vi "clip_max_search.vi"(0 "input cluster":T1, 1 "Channel":i32, 2 "vclip":i32, 5 "Vatt init":i32=4095, 7 "Boolean":bool=TRUE, 9 "Voltage value":dbl=0.05, 11 "error out 2":errorcluster) -> (4 "output cluster":T1={"AWG VISA"="81160A", "Oscilloscope  VISA "="", "Integration Board IP"="172.16.7.43", "connection ID"=refnum, "report out"=refnum, "report file path"=path ""}, 6 "Vatt init":i32, 8 "vclip":i32, 10 "L1 value":i32, 15 "error out":errorcluster)   [LabVIEW 2009]
uses:
  <vilib>/Utility/NIReport.llb/NI_report.lvclass
  <instrlib>/Agilent 81150/Agilent 81150.lvlib
panel:
  in  "vclip_fi":i32
  out "L1 vs vatt":cluster{i32[], i32[]}(graph)
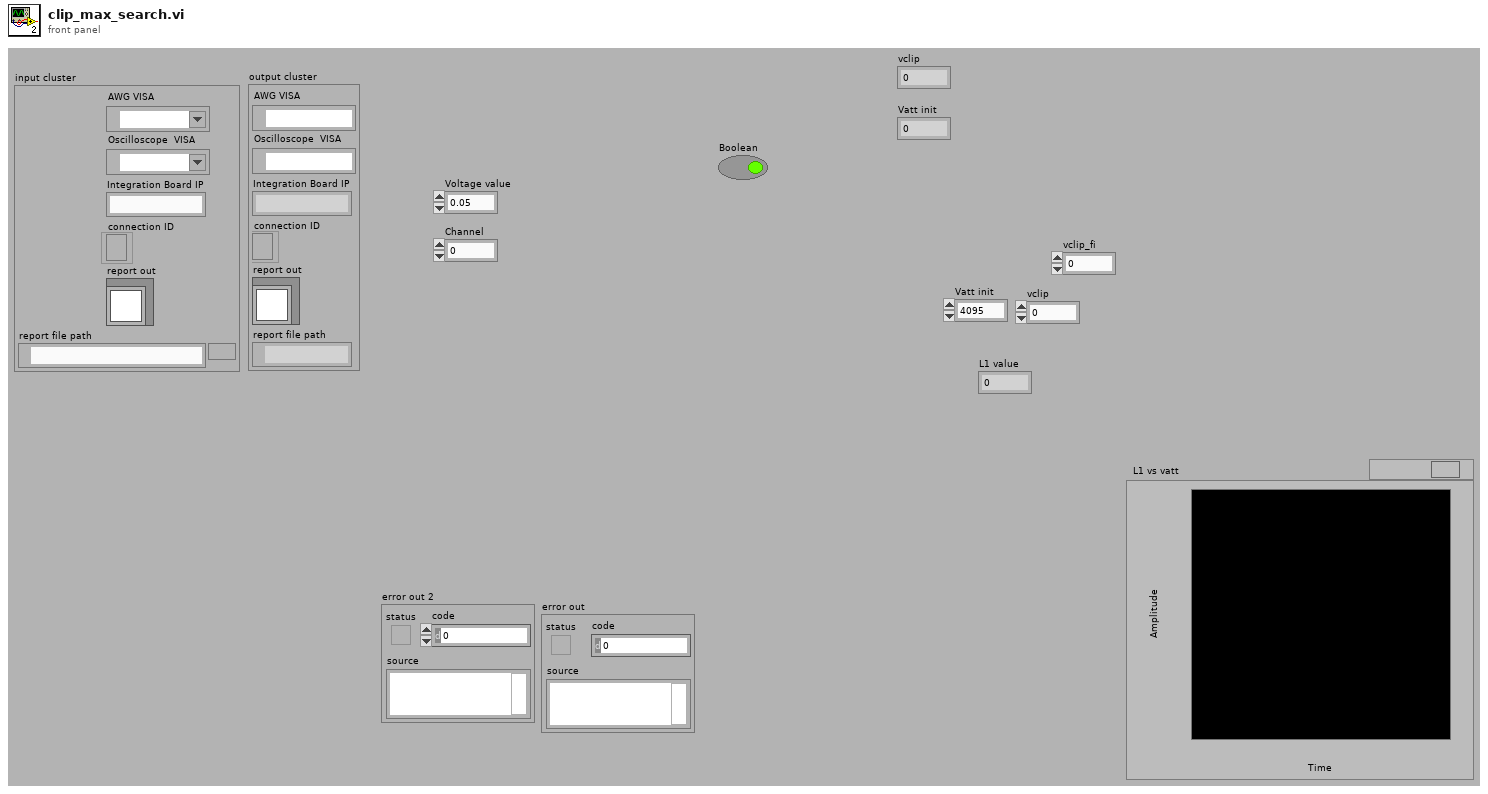
[diagram p1: front panel]
types:
  T1 = cluster{"AWG VISA":refnum<visa-resource-name>, "Oscilloscope  VISA ":refnum<visa-resource-name>, "Integration Board IP":string, "connection ID":refnum<k5>, "report out":refnum<class "NI_report.lvclass">, "report file path":path}
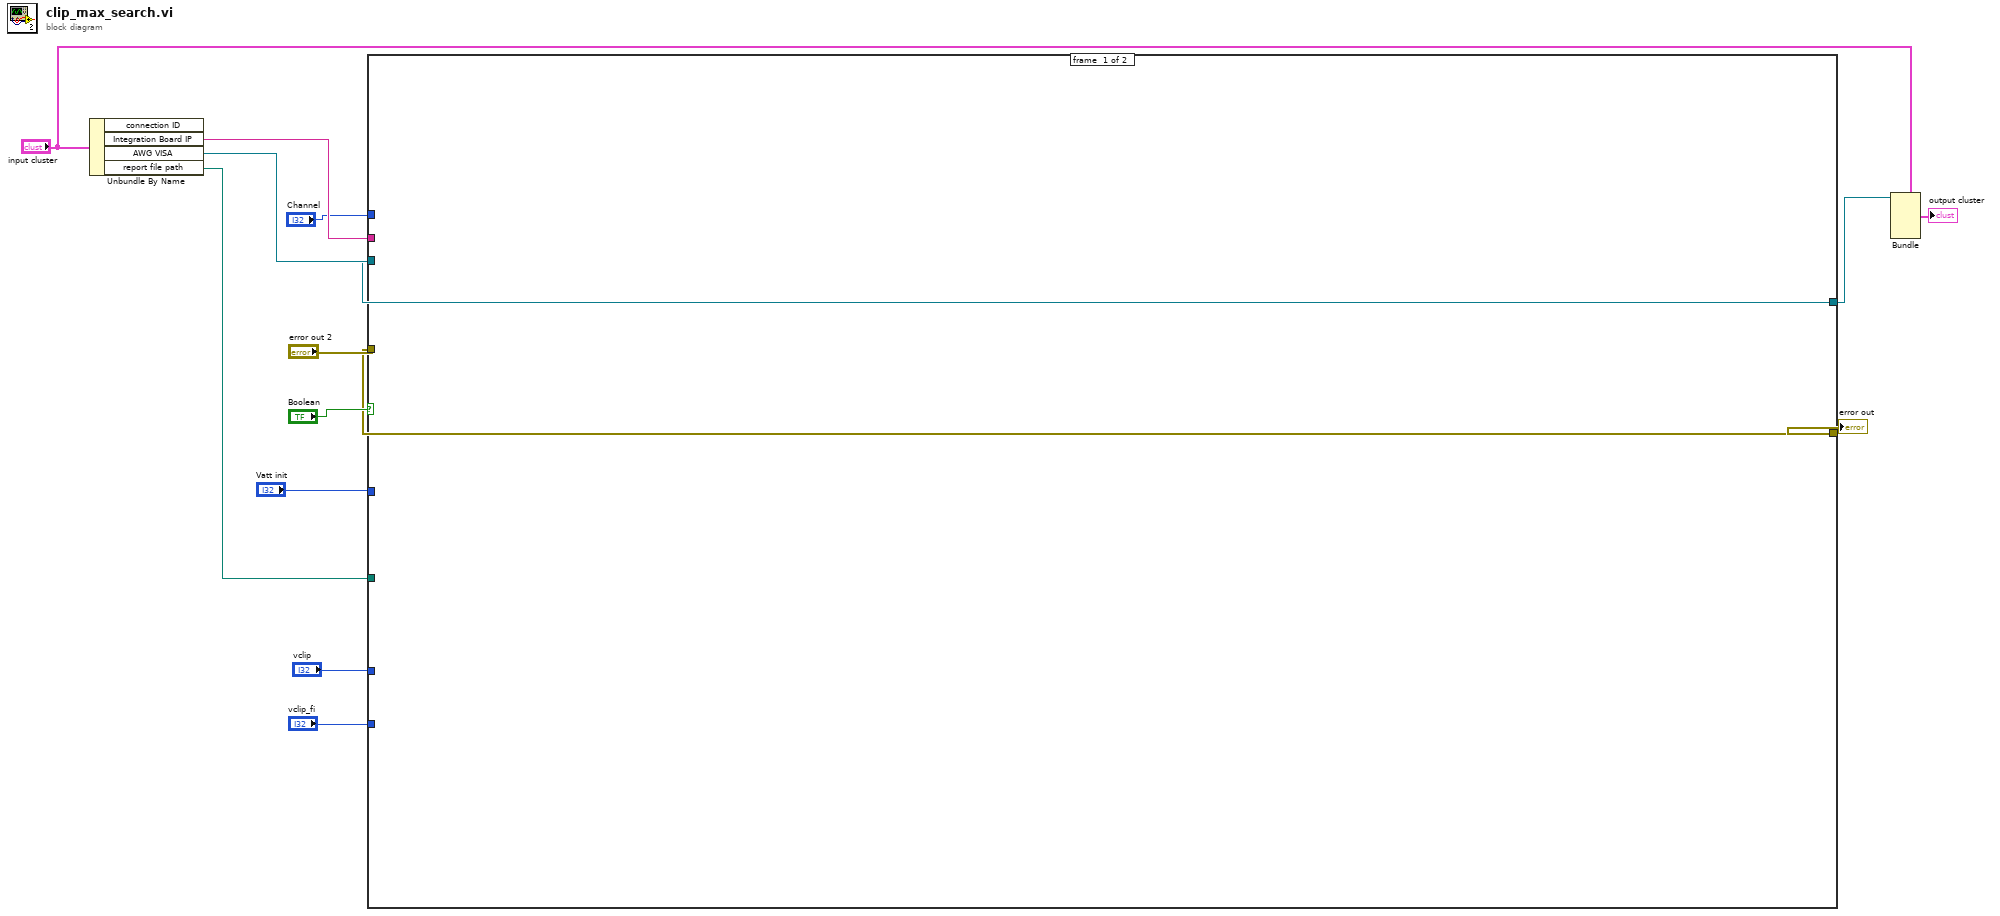
[diagram p0: block diagram]
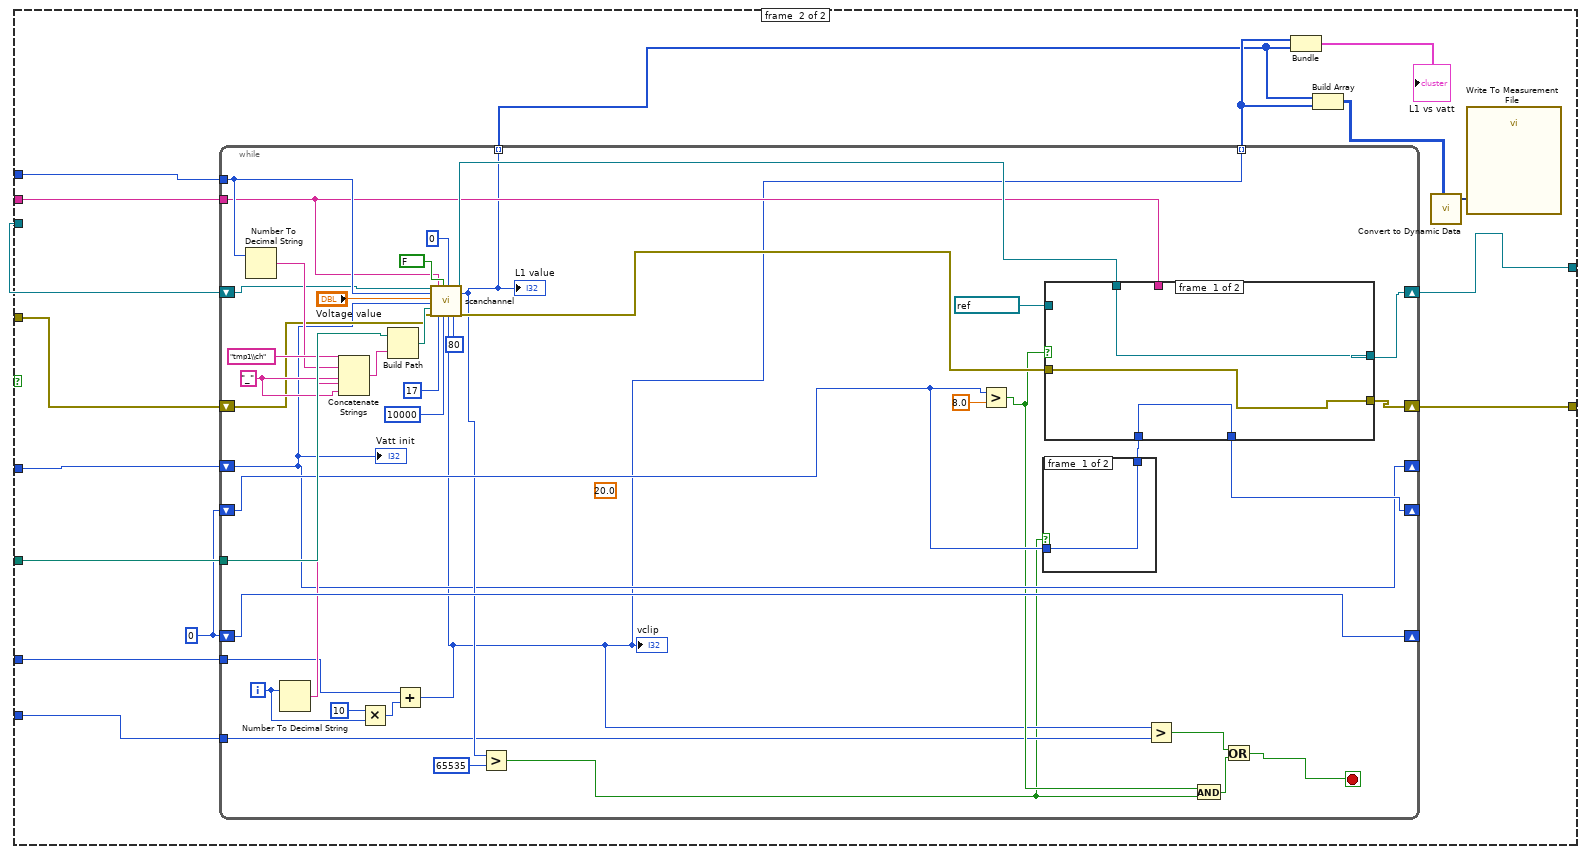
[diagram p2: hidden frame]
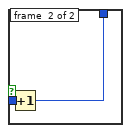
[diagram p3: hidden frame]
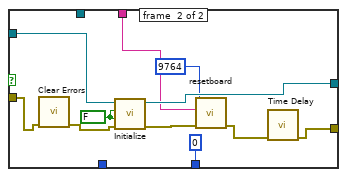
[diagram p4: hidden frame]
diagram:
  n1 = Unbundle By Name("input cluster") -> ("Integration Board IP"=w9:string, "AWG VISA"=w2:refnum<visa-resource-name>, "report file path"=w10:path)  [unwired: 1 out]
  n2 = case shown="True" "Boolean" {
    tunnel: "error out 2" -> [w15 w23]
    tunnel: w9 -> [_ w31]
    tunnel: w10 -> [_ w30]
    tunnel: "vclip" -> [_ w29]
    tunnel: "Vatt init" -> [_ w28]
    tunnel: [w15 w26] -> w13
    tunnel: "Channel" -> [_ w27]
    tunnel: [w14 w24] -> w4
    tunnel: w2 -> [w14 w25]
    tunnel: "vclip_fi" -> [_ w21]
    frame #0 {
    }
    frame #1 {
      w22 = 0
      n3 = while {
        tunnel: w31 -> [w50]
        tunnel: w30 -> [w72]
        shift-right: [w47] -> _
        shift-left: w28 -> [w47]
        shift-right: [w71] -> _
        shift-left: w22 -> [w71]
        tunnel: w27 -> [w60]
        shift-right: [w53] -> w24
        shift-left: w25 -> [w58]
        shift-right: [w55] -> w26
        shift-left: w23 -> [w57]
        shift-right: [w51] -> _
        shift-left: w22 -> [w52]
        tunnel: [w48] -> w18 mode=indexing
        tunnel: [w33] -> w19 mode=indexing
        tunnel: w21 -> [w34]
        tunnel: w29 -> [w39]
        i -> [w41]
        stop <- w36 stop-if-true
        (unwired) 20.0 ("upper limit")
        w61 = "_" ("string")
        n4 = Number To Decimal String(number=w60) -> (decimal integer string=w63:string)  [unwired: 1 in]
        n5 = Number To Decimal String(number=w41) -> (decimal integer string=w62:string)  [unwired: 1 in]
        n6 = Concatenate Strings("tmp1\\ch" ("name or relative path"), w63, w61, w62, w61) -> (w65:string)
        n7 = Multiply(x=10, y=w41) -> (x*y=w38:i32)
        n8 = Build Path(base path=w72, name or relative path=w65) -> (appended path=w70:path)
        n9 = Add(x=w39, y=w38) -> (x+y=w33:i32)
        "vclip" <- w33
        n10 = call "scanchannel.vi"("VISA resource name out"=w58, "num ch"=w60, "Voltage value"="Voltage value", "Init vatt value"=w47, "base path"=w70, "error in"=w57, "Integration Board IP"=w50, "L1 Address"=17 ("Value"), "Save test data"=FALSE, "Ch burst"=10000, "Delay"=0, "vclip"=w33, "initial value"=80) -> ("VISA resource name out 2"=w54:refnum<visa-resource-name>, "L1 value"=w48:i32, "error out"=w56:errorcluster)  [unwired: 4 in]
        "L1 value" <- w48
        n11 = Greater?(x=w48, y=65535) -> (0:w32:bool)
        n12 = Greater?(x=w52, y=8.0) -> (0:w42:bool)
        n13 = case shown="False" w32 {
          tunnel: w52 -> [w73 w75]
          tunnel: [w73 w74] -> w45
          frame #0 {
          }
          frame #1 {
            n14 = Increment(x=w75) -> (x+1=w74:i32)
          }
        }
        n15 = case shown="False" w42 {
          tunnel: w56 -> [w77 w81]
          tunnel: [w77 w85] -> w55
          tunnel: [w78 w89] -> w53
          tunnel: w54 -> [w78 _]
          tunnel: w50 -> [_ w83]
          tunnel: [w76 0] -> w51
          tunnel: w45 -> [w76 _]
          tunnel: refnum<visa-resource-name> "81160A" ("VISA resource name") -> [_ w79]
          frame #0 {
          }
          frame #1 {
            w88 = FALSE ("Reset (True)")
            n16 = call <vilib>:"Clear Errors.vi"("error in (no error)"=w81) -> ("error out"=w80:errorcluster)  [unwired: 6 in]
            n17 = call <instrlib>:"Initialize.vi"("error in (no error)"=w80, "Reset (True)"=w88, "ID Query (True)"=w88, "VISA resource name"=w79) -> ("error out"=w87:errorcluster, "VISA resource name out"=w89:refnum<visa-resource-name>)  [unwired: 6 in]
            n18 = call "resetboard.vi"("error in (no error)"=w87, "address"=w83, "remote port or service name"=u16 9764) -> ("error out"=w86:errorcluster)  [unwired: 7 in, 1 out]
            n19 = call "Time Delay"("error in (no error)"=w86) -> ("error out"=w85:errorcluster)  [unwired: 10 in]
          }
        }
        n20 = Greater?(x=w33, y=w34) -> (0:w35:bool)
        n21 = And(x=w42, y=w32) -> (x .and. y?=w37:bool)
        n22 = Or(x=w35, y=w37) -> (x .or. y?=w36:bool)
        "Vatt init" <- w47
      }
      n23 = Bundle(w19, w18) -> (→"L1 vs vatt":cluster{i32[], i32[]})  [unwired: 1 in]
      n24 = Build Array(w18, w19) -> (w17:i32[][])
      n25 = call "Convert to Dynamic Data"("2D Array"=w17) -> ("Dynamic Data Type"=w16:dynamicdata)  [unwired: 3 in]
      n26 = call "Write To Measurement File"("Signals"=w16) -> ()  [unwired: 16 in, 3 out]
    }
  }
  "error out" <- w13
  n27 = Bundle(cluster="input cluster", "AWG VISA"=w4) -> (→"output cluster":T1)  [unwired: 5 in]
